vi "init.vi"(8 "error in":errorcluster, 10 "component configuration":refnum<class "TBM module configuration.lvclass">, 11 "asynchronous execution module runtime In":refnum<class "asynchronous execution module runtime.lvclass">) -> (0 "error out":errorcluster, 1 "data allocations":T1, 2 "execution settings":T4, 3 "asynchronous execution module runtime Out":refnum<class "asynchronous execution module runtime.lvclass">)   [LabVIEW 2013, in "asynchronous execution module runtime.lvclass"]
doc: "Provides an interface for initializing a component at runtime. While this interface performs no operations, a child should provide an override which may open any necessary references or sessions, allocate necessary memory, and perform any final configuration validataion before providing the full configuration <b>execution data</b> to the calling process."
uses:
  asynchronous execution module runtime.lvclass
  <vilib>/NI/Tag Bus Module Framework/module configuration/TBM module configuration.lvclass
  <vilib>/NI/Tag Bus Module Framework/runtime/execution settings.ctl
  <vilib>/NI/Tag Bus Module Framework/channel/data tables.ctl
  <vilib>/NI/Tag Bus/dictionary/data dictionary.lvclass
  <vilib>/NI/Tag Bus/dictionary table pair.ctl
  <vilib>/NI/Tag Bus/table/data table.ctl
  configuration/asynchronous execution module configuration.lvclass
  <vilib>/NI/Tag Bus Module Framework/runtime/TBM module execution interface.lvclass
  Framework Configuration Classes/platypus configuration/class discovery singleton methods.ctl
  configuration/asynchronous execution module configuration.lvclass/asynchronous execution module configuration.ctl
  asynchronous execution module runtime.lvclass/asynchronous execution module runtime.ctl
  Framework Configuration Classes/platypus configuration/PLConfigurationSerializer.lvlib
  <vilib>/NI/Tag Bus/tag bus.lvlib
  <vilib>/NI/Tag Bus Module Framework/channel/TBM channel.lvclass
  <vilib>/NI/Tag Bus/table/data table.lvlib
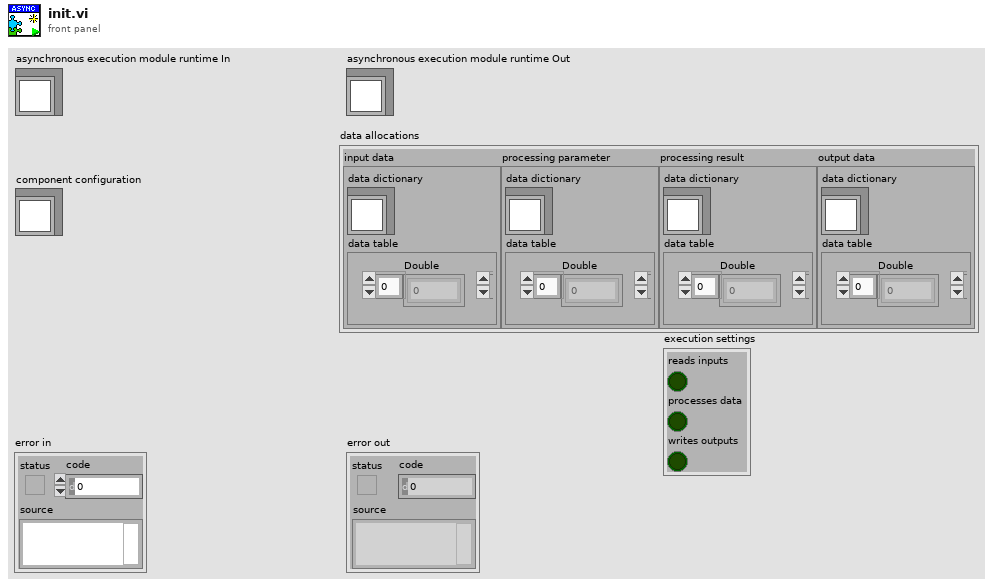
[diagram p1: front panel]
types:
  T1 = typedef "TBM channel.lvclass/data tables.ctl" = cluster{"input data":T2, "processing parameter":T2, "processing result":T2, "output data":T2}
  T2 = typedef "tag bus.lvlib/dictionary table pair.ctl" = cluster{"data dictionary":refnum<class "data dictionary.lvclass">, "data table":T3}
  T3 = typedef "tag bus.lvlib/data table.lvlib/data table.ctl" = cluster{"Double":dbl[], "Single":sgl[], "I64":i64[], "I32":i32[], "I16":i16[], "I8":i8[], "U64":u64[], "U32":u32[], "U16":u16[], "U8":u8[], "Boolean":bool[], "String":string[], "Array of Double":cluster{"DBL Array":dbl[]}[], "Array of Single":cluster{"SGL Array":sgl[]}[], "Array of I64":cluster{"I64 Array":i64[]}[], "Array of I32":cluster{"I32 Array":i32[]}[], "Array of I16":cluster{"I16 Array":i16[]}[], "Array of I8":cluster{"I8 Array":i8[]}[], "Array of U64":cluster{"U64 Array":u64[]}[], "Array of U32":cluster{"U32 Array":u32[]}[], "Array of U16":cluster{"U16 Array":u16[]}[], "Array of U8":cluster{"U8 Array":u8[]}[], "Array of Boolean":cluster{"Boolean Array":bool[]}[], "Array of String":cluster{"String Array":string[]}[]}
  T4 = typedef "TBM module execution interface.lvclass/execution settings.ctl" = cluster{"reads inputs":bool, "processes data":bool, "writes outputs":bool}
  T5 = typedef "PLConfigurationSerializer.lvlib/class discovery singleton methods.ctl" = enum16{"add search paths", "load class by name"}
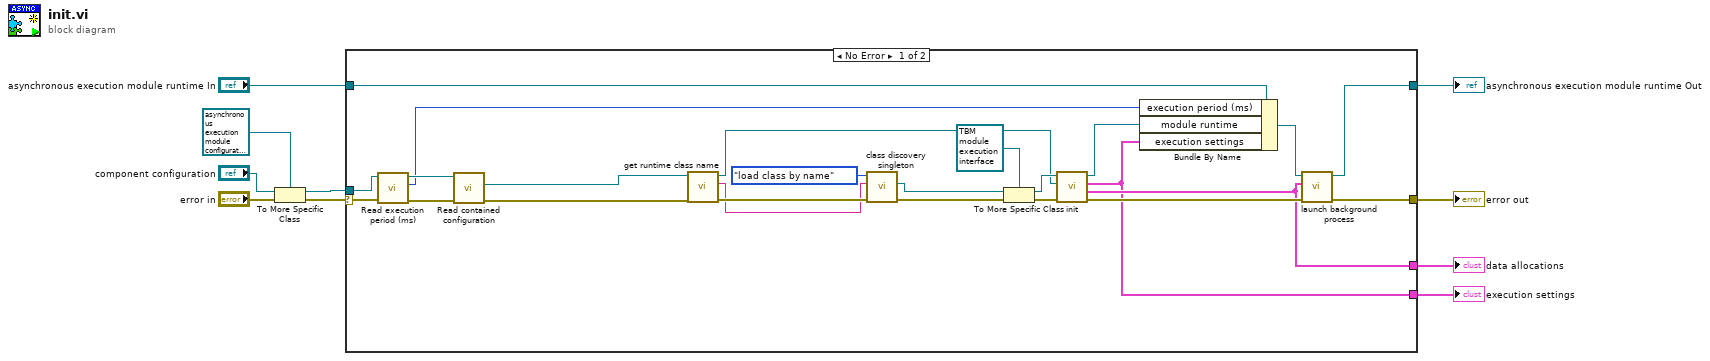
[diagram p0: block diagram]
diagram:
  n1 = To More Specific Class(target class=refnum<class "asynchronous execution module configuration.lvclass"> refnum ("CVT Access Configuration"), reference="component configuration", error in="error in") -> (specific class reference=w6:refnum<class "asynchronous execution module configuration.lvclass">, error out=w7:errorcluster)
  n2 = case shown="No Error" w7 {
    selector: w7 -> [w17 w35]
    tunnel: w6 -> [w15 _]
    tunnel: "asynchronous execution module runtime In" -> [w34 w36]
    tunnel: [w31 w36] -> w4
    tunnel: [w33 w35] -> w3
    tunnel: [w21 _] -> w2
    tunnel: [w25 _] -> w1
    frame No Error {
      n3 = call "Read execution period (ms).vi"("error in"=w17, "Asynchronous Component Configuration in"=w15) -> ("error out"=w16:errorcluster, "execution period (ms)"=w13:i32, "Asynchronous Component Configuration out"=w14:refnum<class "asynchronous execution module configuration.lvclass">)  [unwired: 7 in]
      n4 = call "Read contained configuration.vi"("error in"=w16, "asynchronous execution module configuration in"=w14) -> ("error out"=w11:errorcluster, "module configuration"=w12:refnum<class "TBM module configuration.lvclass">)  [unwired: 7 in, 1 out]
      n5 = call-dynamic "get runtime class name.vi"("error in"=w11, "module configuration in"=w12) -> ("error out"=w19:errorcluster, "class name"=w18:string, "module configuration out"=w20:refnum<class "TBM module configuration.lvclass">)  [unwired: 7 in]
      n6 = call "class discovery singleton.vi"("error in"=w19, "Class Name"=w18, "method"=class_discovery_singleton_methods."load class by name") -> ("error out"=w24:errorcluster, "LabVIEW Object"=w23:refnum<class>)  [unwired: 7 in]
      n7 = To More Specific Class(target class=refnum<class "TBM module execution interface.lvclass"> refnum ("Component Runtime Interface"), reference=w23, error in=w24) -> (specific class reference=w28:refnum<class "TBM module execution interface.lvclass">, error out=w29:errorcluster)
      n8 = call-dynamic "init.vi"("error in"=w29, "module configuration"=w20, "module in"=w28) -> ("error out"=w26:errorcluster, "data allocations"=w25:T1, "execution settings"=w21:T4, "module out"=w27:refnum<class "TBM module execution interface.lvclass">)  [unwired: 5 in]
      n9 = Bundle By Name(cluster=w34, "execution period (ms)"=w13, "module runtime"=w27, "execution settings"=w21) -> (w32:refnum<class "asynchronous execution module runtime.lvclass">)
      n10 = call "launch background process.vi"("error in"=w26, "data allocations"=w25, "asynchronous execution module runtime In"=w32) -> ("error out"=w33:errorcluster, "asynchronous execution module runtime Out"=w31:refnum<class "asynchronous execution module runtime.lvclass">)  [unwired: 7 in]
    }
    frame Error {
    }
  }
  "error out" <- w3
  "asynchronous execution module runtime Out" <- w4
  "execution settings" <- w2
  "data allocations" <- w1
